vi "Point-in-Box test (object-oriented).vi"(1 "Point":sgl[](array[numeric]), 2 "Box":T1) -> (0 "Point is inside box":bool)   [LabVIEW 2014]
uses:
  Typedefs/TreeNodeBox.ctl
  Typedefs/Quad.ctl
  Typedefs/Quadplane enum.ctl
panel:
  # "PN 17/01/2015"
  # "Vertices"
  # "Edges"
  # "Unit normal"
  # "Plane ident."
  # "Vertices"
  # "Edges"
  # "Unit normal"
  # "Plane ident."
  # "Vertices"
  # "Edges"
  # "Unit normal"
  # "Plane ident."
  # "Vertices"
  # "Edges"
  # "Unit normal"
  # "Plane ident."
  # "Vertices"
  # "Edges"
  # "Unit normal"
  # "Plane ident."
  # "Vertices"
  # "Edges"
  # "Unit normal"
  # "Plane ident."
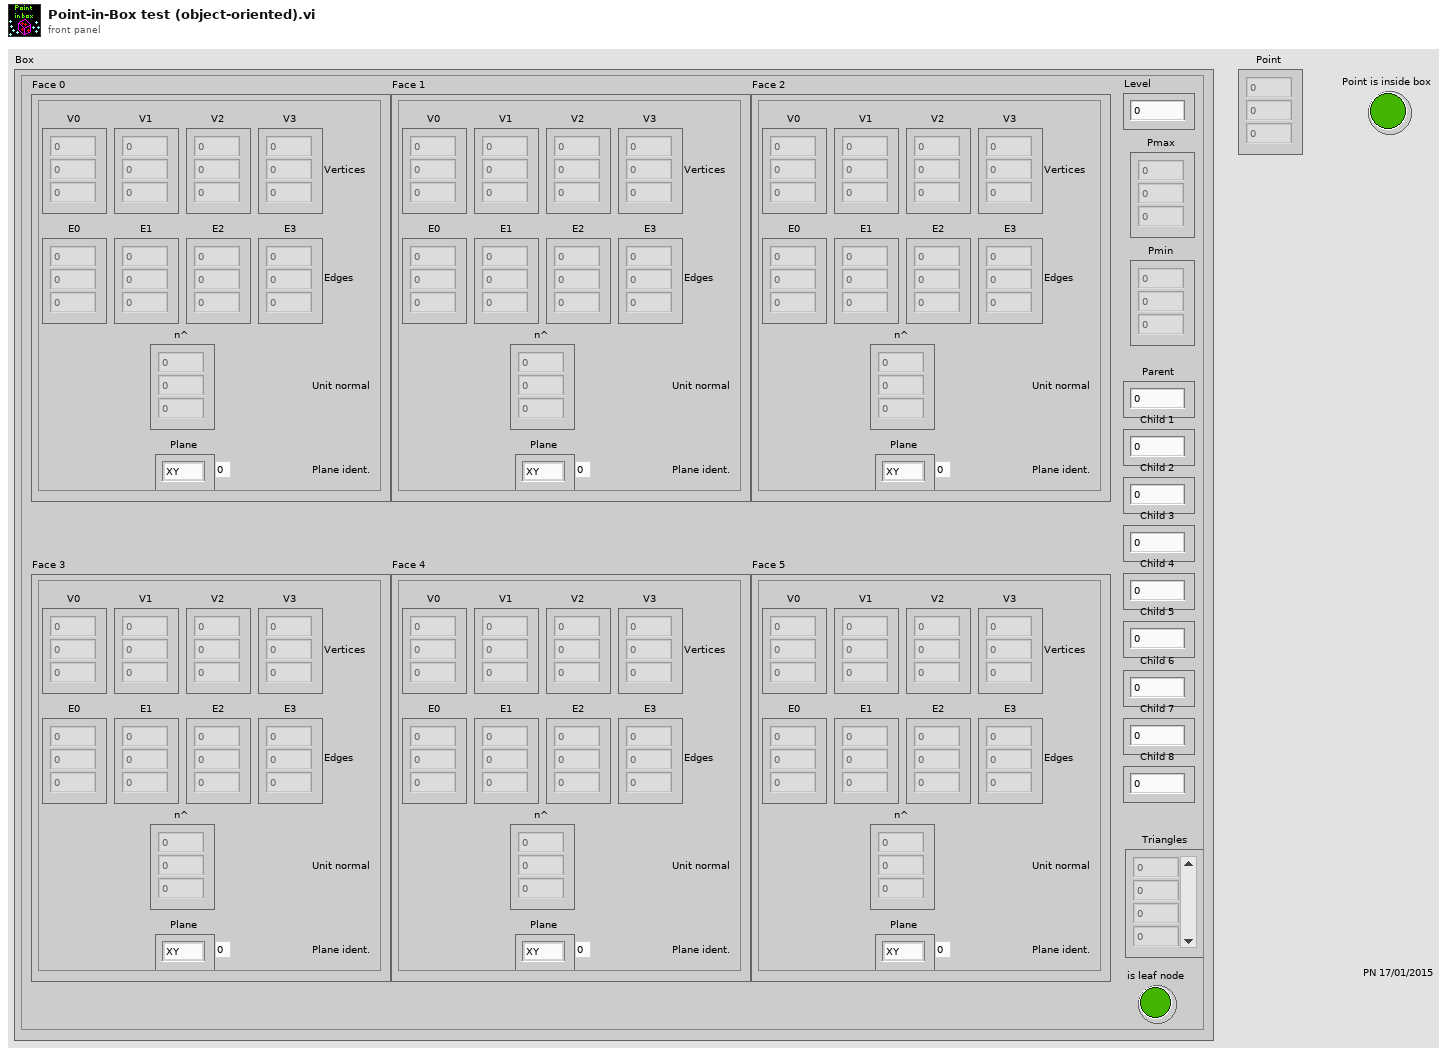
[diagram p1: front panel]
types:
  T1 = typedef "TreeNodeBox.ctl" = cluster{"Face 0":T2, "Face 1":T2, "Face 2":T2, "Face 3":T2, "Face 4":T2, "Face 5":T2, "Level":i32, "Pmax":sgl[], "Pmin":sgl[], "Parent":i32, "Child 1":i32, "Child 2":i32, "Child 3":i32, "Child 4":i32, "Child 5":i32, "Child 6":i32, "Child 7":i32, "Child 8":i32, "Triangles":i32[], "is leaf node":bool}
  T2 = typedef "Quad.ctl" = cluster{"V0":sgl[], "V1":sgl[], "V2":sgl[], "V3":sgl[], "E0":sgl[], "E1":sgl[], "E2":sgl[], "E3":sgl[], "n^":sgl[], "Plane":T3}
  T3 = typedef "Quadplane enum.ctl" = enum8{"XY", "XZ", "YZ", "-XY", "-XZ", "-YZ"}
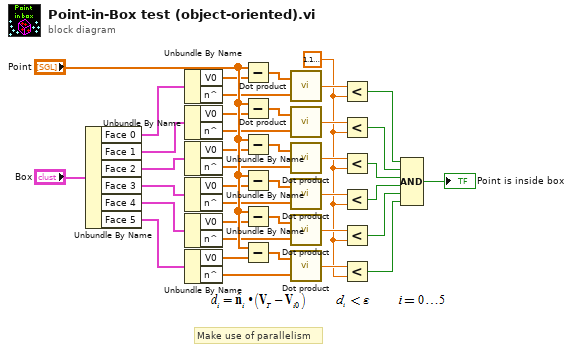
[diagram p0: block diagram]
diagram:
  w8 = sgl 1.1920929e-07
  # "Make use of parallelism"
  n1 = Unbundle By Name("Box") -> ("Face 0"=w39:T2, "Face 1"=w38:T2, "Face 2"=w37:T2, "Face 3"=w36:T2, "Face 4"=w35:T2, "Face 5"=w34:T2)
  n2 = Unbundle By Name(w39) -> ("V0"=w32:sgl[], "n^"=w26:sgl[])
  n3 = Unbundle By Name(w38) -> ("V0"=w31:sgl[], "n^"=w19:sgl[])
  n4 = Unbundle By Name(w37) -> ("V0"=w30:sgl[], "n^"=w18:sgl[])
  n5 = Unbundle By Name(w36) -> ("V0"=w29:sgl[], "n^"=w17:sgl[])
  n6 = Unbundle By Name(w35) -> ("V0"=w28:sgl[], "n^"=w16:sgl[])
  n7 = Unbundle By Name(w34) -> ("V0"=w27:sgl[], "n^"=w15:sgl[])
  n8 = Subtract(x="Point", y=w32) -> (x-y=w25:sgl[])
  n9 = Subtract(x="Point", y=w31) -> (x-y=w24:sgl[])
  n10 = Subtract(x="Point", y=w30) -> (x-y=w23:sgl[])
  n11 = Subtract(x="Point", y=w29) -> (x-y=w22:sgl[])
  n12 = Subtract(x="Point", y=w28) -> (x-y=w21:sgl[])
  n13 = Subtract(x="Point", y=w27) -> (x-y=w20:sgl[])
  n14 = call "Dot product.vi"("B"=w26, "A"=w25) -> ("A . B"=w14:sgl)
  n15 = call "Dot product.vi"("B"=w19, "A"=w24) -> ("A . B"=w13:sgl)
  n16 = call "Dot product.vi"("B"=w18, "A"=w23) -> ("A . B"=w12:sgl)
  n17 = call "Dot product.vi"("B"=w17, "A"=w22) -> ("A . B"=w11:sgl)
  n18 = call "Dot product.vi"("B"=w16, "A"=w21) -> ("A . B"=w10:sgl)
  n19 = call "Dot product.vi"("B"=w15, "A"=w20) -> ("A . B"=w9:sgl)
  n20 = Less?(x=w14, y=w8) -> (x < y?=w7:bool)
  n21 = Less?(x=w13, y=w8) -> (x < y?=w6:bool)
  n22 = Less?(x=w12, y=w8) -> (x < y?=w5:bool)
  n23 = Less?(x=w11, y=w8) -> (x < y?=w4:bool)
  n24 = Less?(x=w10, y=w8) -> (x < y?=w3:bool)
  n25 = Less?(x=w9, y=w8) -> (x < y?=w2:bool)
  n26 = Compound Arithmetic op=AND(w7, w6, w5, w4, w3, w2) -> (→"Point is inside box":bool)
